vi "Get Set FGV.vi"(7 "Method (Get)":enum16{"Get", "Set"}(ring), 8 "error in":errorcluster, 10 "Data In":variant, 11 "Name":string) -> (0 "error out":errorcluster, 3 "Data out":variant)   [LabVIEW 2021]
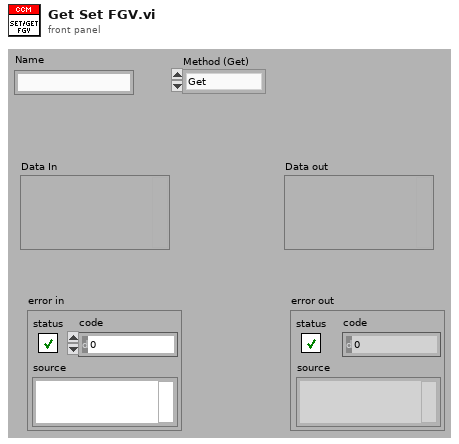
[diagram p1: front panel]
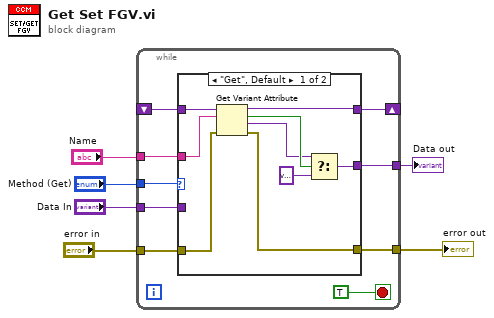
[diagram p0: block diagram]
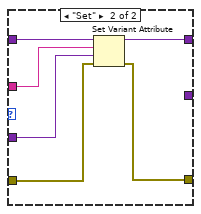
[diagram p2: hidden frame]
diagram:
  n1 = while {
    tunnel: "Method (Get)" -> [w15]
    tunnel: "Name" -> [w12]
    shift-right: [w13] -> _
    shift-left: _ -> [w14]
    tunnel: [w10] -> w4
    tunnel: "Data In" -> [w9]
    tunnel: "error in" -> [w8]
    tunnel: [w7] -> w2
    stop <- TRUE stop-if-true
    n2 = case shown="\"Get\", Default" w15 {
      tunnel: w9 -> [_ w27]
      tunnel: w14 -> [w24 w30]
      tunnel: [w23 w29] -> w13
      tunnel: w12 -> [w22 w28]
      tunnel: [w19 _] -> w10
      tunnel: w8 -> [w17 w26]
      tunnel: [w16 w25] -> w7
      frame "Get", Default {
        n3 = Get Variant Attribute(Variant=w24, name=w22, error in=w17) -> (duplicate Variant=w23:variant, found=w21:bool, value=w20:variant, error out=w16:errorcluster)  [unwired: 1 in]
        n4 = Select(t=w20, s=w21, f=variant) -> (s? t:f=w19:variant)
      }
      frame "Set" {
        n5 = Set Variant Attribute(Variant=w30, name=w28, value=w27, error in=w26) -> (Variant out=w29:variant, error out=w25:errorcluster)  [unwired: 1 out]
      }
    }
  }
  "error out" <- w2
  "Data out" <- w4
